vi "Create Async.vi"() -> ()   [LabVIEW 2021, in "Q Async.lvlib"]
uses:
  Q Async.lvlib
  Loop.vi
panel:
  in  "Numeric":i32=4
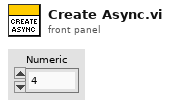
[diagram p1: front panel]
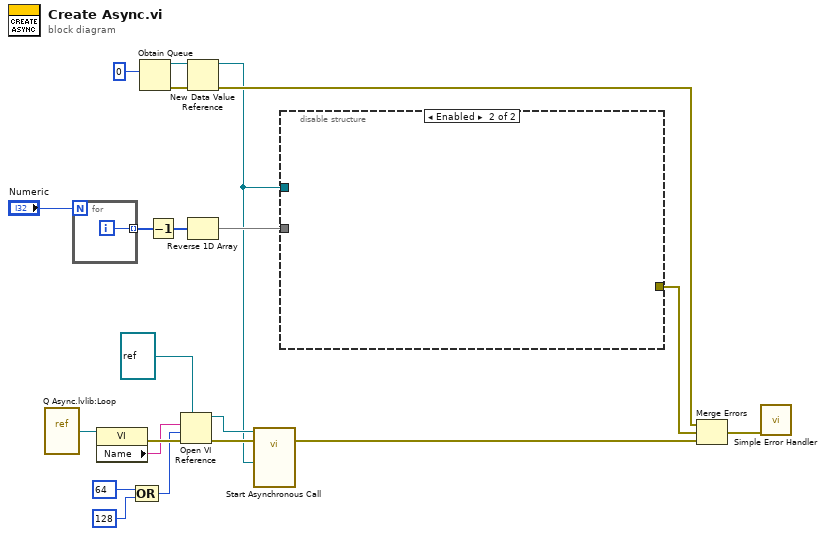
[diagram p0: block diagram]
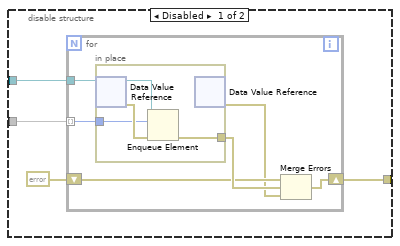
[diagram p2: hidden frame]
diagram:
  n1 = vi-ref "Q Async.lvlib:Loop.vi"() -> (w10:refnum<vi>)
  n2 = for {
    N: "Numeric" -> [_]
    tunnel: [w22] -> w20 mode=indexing
    i -> [w22]
  }
  n3 = property class="VI"(reference=w10) -> (error out=w9:errorcluster, "Name"=w8:string)  [unwired: 1 in, 1 out]
  n4 = Compound Arithmetic op=OR(64 ("options"), 128 ("options")) -> (w5:i32)
  n5 = Obtain Queue(element data type=0) -> (queue out=w18:refnum<queue>, error out=w15:errorcluster)  [unwired: 4 in, 1 out]
  n6 = Decrement(x=w20) -> (x-1=w21:i32[])
  n7 = Open VI Reference(type specifier VI Refnum (for type only)=refnum<vi> refnum, vi path=w8, options=w5, error in (no error)=w9) -> (vi reference=w2:refnum<vi>, error out=w3:errorcluster)  [unwired: 2 in]
  n8 = New Data Value Reference(data value=w18, error in=w15) -> (data value reference=w1:refnum<data-value>, error out=w12:errorcluster)
  n9 = Reverse 1D Array(array=w21) -> (reversed array=w16:i32[])
  n10 = call-by-ref "Start Asynchronous Call"(reference=w2, error in=w3, "DVR"=w1) -> (error out=w4:errorcluster)  [unwired: 11 in, 1 out]
  n11 = disable-structure shown="Enabled" {
    disable-tunnel: w16 -> [w26 _]
    disable-tunnel: [w24 _] -> w14
    disable-tunnel: w1 -> [w23 _]
    frame Disabled {
      n12 = for {
        tunnel: w23 -> [w32]
        tunnel: w26 -> [w31] mode=indexing
        shift-right: [w29] -> w24
        shift-left: errorcluster {"status"=FALSE, "code"=0, "source"=""} ("error out") -> [w28]
        n13 = in-place {
          in-place-border: w31 -> [w33]
          in-place-border: [w34] -> w30
          n14 = in-place-dvr #1(w32) -> (w36:refnum<queue>, w35:errorcluster)
          n15 = Enqueue Element(queue=w36, element=w33, error in (no error)=w35) -> (error out=w34:errorcluster)  [unwired: 1 in, 2 out]
          n16 = in-place-dvr #1() -> (w27:errorcluster)  [unwired: 1 in, 1 out]
        }
        n17 = Merge Errors(w28, w30, w27) -> (w29:errorcluster)
      }
    }
    frame Enabled {
    }
  }
  n18 = Merge Errors(w12, w14, w4) -> (w13:errorcluster)
  n19 = call <vilib>:"Simple Error Handler.vi"("error in (no error)"=w13) -> ()  [unwired: 4 in, 5 out]
